vi "Read HWS file and Convert to Data.vi"(7 "Register Address":u8=28 format="%.0x", 11 "Starting HWS File":path=path "C:/Users/er080167/Documents/XP2100/Waveforms/BRGu8r1Cd57.hws") -> (3 "Converted Data":T1 {"Register" max=31 format="%.0x"; "Slave Address" max=15 format="%.0x"})   [LabVIEW 2013]
uses:
  <vilib>/Waveform/DTblOps.llb/DTbl Digital to Boolean Array.vi
panel:
  out "HWS File Read":digitalwaveform(graph)
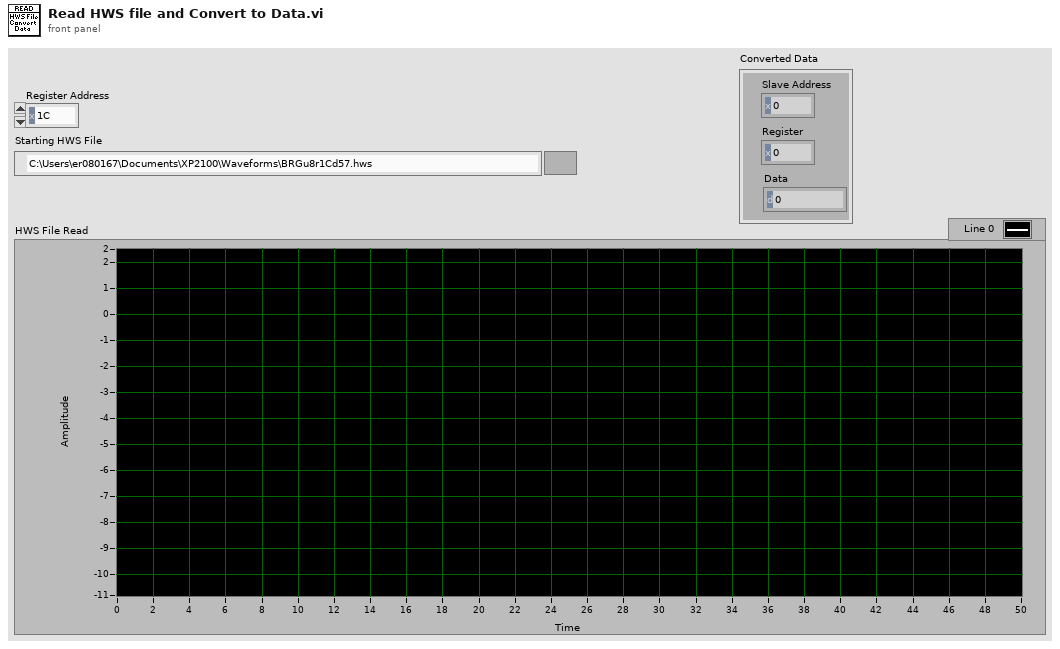
[diagram p1: front panel]
types:
  T1 = cluster{"Slave Address":u8, "Register":u8, "Data":u8}
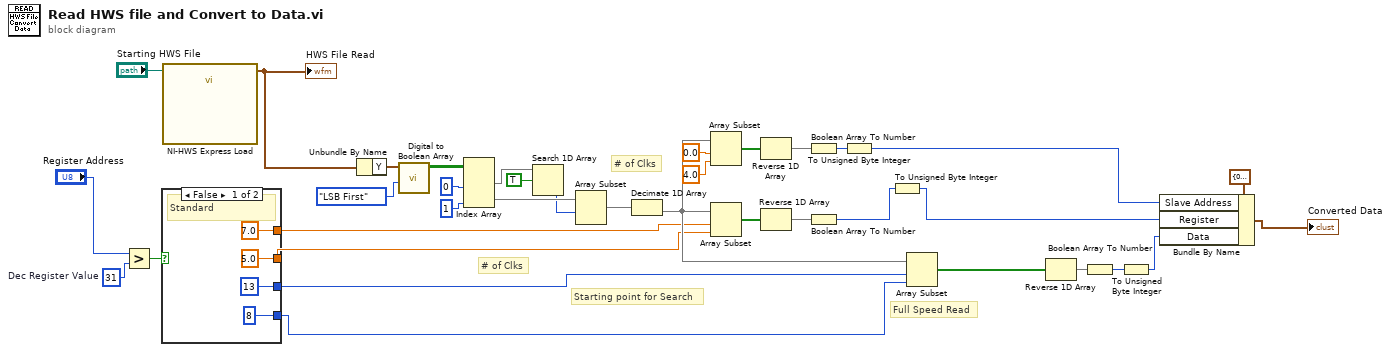
[diagram p0: block diagram]
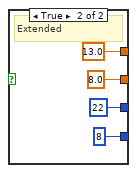
[diagram p2: hidden frame]
diagram:
  w10 = u8 31  # Dec Register Value
  # "Full Speed Read"
  # "Starting point for Search"
  # "# of Clks"
  # "# of Clks"
  n1 = Greater?(x="Register Address", y=w10) -> (0:w9:bool)
  n2 = case shown="False" w9 {
    tunnel: [7.0 ("input variable") 13.0 ("input variable")] -> w8
    tunnel: [5.0 ("input variable") 8.0 ("input variable")] -> w7
    tunnel: [13 ("start index (0)") 22 ("start index (0)")] -> w5
    tunnel: [8 ("length") 8 ("length")] -> w6
    frame False {
      # "Standard"
    }
    frame True {
      # "Extended"
    }
  }
  n3 = call "NI-HWS Express Load"("file path"="Starting HWS File") -> ("EnableOdft.hws"=w2:digitalwaveform)  [unwired: 9 in, 1 out]
  "HWS File Read" <- w2
  n4 = Unbundle By Name(w2) -> ("Y"=w27:digitaldata)
  n5 = call-poly <vilib>:"Digital to Boolean Array.vi"("mode"=enum16{"LSB First", "MSB First"}."LSB First", "digital data"=w27) -> ("boolean array"=w33:bool[][])  [unwired: 8 in, 1 out]
  n6 = Index Array(array=w33, index (col) #1=0 ("disabled index (col)"), index (col) #2=1 ("index (col)")) -> (element #1=w26:bool[], element #2=w25:bool[])  [unwired: 2 in]
  n7 = Search 1D Array(1D array=w26, element=TRUE) -> (index of element=w4:i32)  [unwired: 1 in]
  n8 = Array Subset(array=w25, index=w4) -> (w22:bool[])  [unwired: 1 in]
  n9 = Decimate 1D Array(w22) -> (w14:bool[])  [unwired: 1 out]
  n10 = Array Subset(array=w14, index=0.0 ("input variable"), length=4.0 ("input variable")) -> (w21:bool[])
  n11 = Array Subset(array=w14, index=w8, length=w7) -> (w19:bool[])
  n12 = Reverse 1D Array(array=w21) -> (reversed array=w20:bool[])
  n13 = Reverse 1D Array(array=w19) -> (reversed array=w18:bool[])
  n14 = Boolean Array To Number(Boolean array=w20) -> (number=w30:u32)
  n15 = Boolean Array To Number(Boolean array=w18) -> (number=w17:u32)
  n16 = To Unsigned Byte Integer(number=w30) -> (unsigned 8bit integer=w28:u8)
  n17 = To Unsigned Byte Integer(number=w17) -> (unsigned 8bit integer=w16:u8)
  n18 = Array Subset(array=w14, index=w5, length=w6) -> (w11:bool[])
  n19 = Reverse 1D Array(array=w11) -> (reversed array=w15:bool[])
  n20 = Boolean Array To Number(Boolean array=w15) -> (number=w13:u32)
  n21 = To Unsigned Byte Integer(number=w13) -> (unsigned 8bit integer=w12:u8)
  n22 = Bundle By Name(cluster=T1 {"Slave Address"=0, "Register"=0, "Data"=0} ("Write Data"), "Slave Address"=w28, "Register"=w16, "Data"=w12) -> (→"Converted Data":T1)
